vi "Intake Immediate with Deadband.vi"(7 "Description":string, 8 "Command Info In":T1, 9 "Deadband Value":dbl=0.01, 10 "Intake Setpoint":dbl) -> (0 "Command Info Out":T1)   [LabVIEW 2019]
doc: "This template includes code for deadband comparision to avoid excessive command scheduling. It is particularly useful for joystick-driven commands.\n\nBe sure to right-click and select New from Template and save with a new command name."
uses:
  <vilib>/Rock Robotics/WPI/Framework/Command Status Info.ctl
  <vilib>/Rock Robotics/WPI/Framework/Completion Status.ctl
  <vilib>/Rock Robotics/WPI/Framework/Completion Notifier.ctl
  Implementation/Intake Setpoints.ctl
  Implementation/Intake Operations.ctl
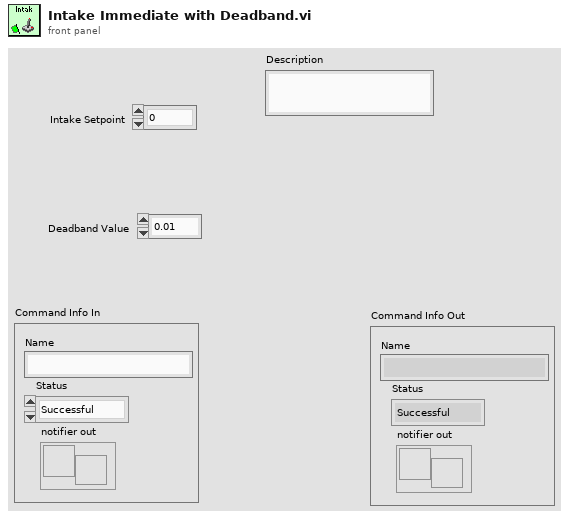
[diagram p1: front panel]
types:
  T1 = typedef "Command Status Info.ctl" = cluster{"Name":string, "Status":T2, "notifier out":T3}
  T2 = typedef "Completion Status.ctl" = enum16{"Successful", "Aborted", "Incomplete"}
  T3 = typedef "Completion Notifier.ctl" = refnum<notifier>
  T4 = typedef "Intake Setpoints.ctl" = cluster{"Operation":T5, "Duration":dbl, "Intake Setpoint":dbl}
  T5 = typedef "Intake Operations.ctl" = enum16{"Reserve", "Read Current", "Immediate", "Change Intake State"}
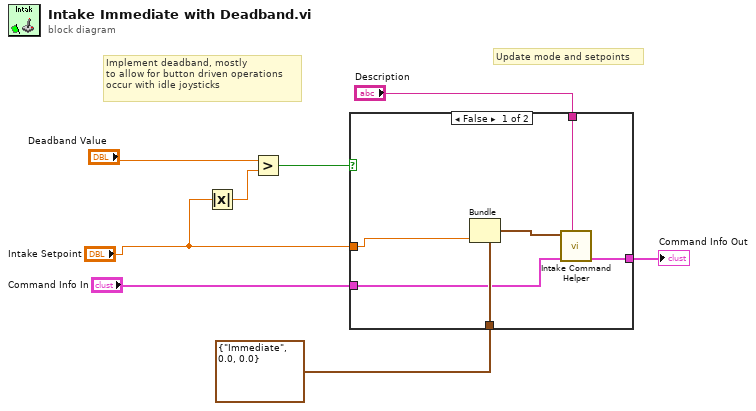
[diagram p0: block diagram]
diagram:
  # "Implement deadband, mostly\nto allow for button driven operations\noccur with idle joysticks"
  # "Update mode and setpoints"
  n1 = Absolute Value(x="Intake Setpoint") -> (abs(x)=w7:dbl)
  n2 = Greater?(x="Deadband Value", y=w7) -> (0:w2:bool)
  n3 = case shown="False" w2 {
    tunnel: T4 {"Operation"=enum."Immediate", "Duration"=0.0, "Intake Setpoint"=0.0} ("SubSystem Data") -> [w14 _]
    tunnel: [w13 w15] -> w6
    tunnel: "Command Info In" -> [w12 w15]
    tunnel: "Description" -> [w10 _]
    tunnel: "Intake Setpoint" -> [w9 _]
    frame False {
      n4 = Bundle(cluster=w14, "Intake Setpoint"=w9) -> (w11:T4)  [unwired: 2 in]
      n5 = call "Intake Command Helper.vi"("Description"=w10, "Command Info In"=w12, "SubSystem Data"=w11) -> ("Command Info Out"=w13:T1)  [unwired: 6 in, 2 out]
    }
    frame True {
    }
  }
  "Command Info Out" <- w6
